vi "Harmonic Power.vi"(8 "error in (no error)":errorcluster, 10 "current spectra":T2(array[cluster]), 11 "voltage spectra":T2(array[cluster])) -> (0 "error out":errorcluster, 1 "total power value":T1, 2 "power values":T1[](array[typedef]), 3 "harmonic power values":T1[][](array[typedef]))   [LabVIEW 2013, in "NI_EP_Power Measurement.lvlib"]
doc: "Calculates the harmonic power values from the phase voltage spectra and the current spectra."
uses:
  <vilib>/addons/Electrical Power/Power Measurement/NI_EP_Power Measurement.lvlib
  <vilib>/addons/Electrical Power/Basic/Measurement/subVIs/basic_Power Value.ctl
  <vilib>/addons/Electrical Power/Basic/NI_EP_Basic.lvlib
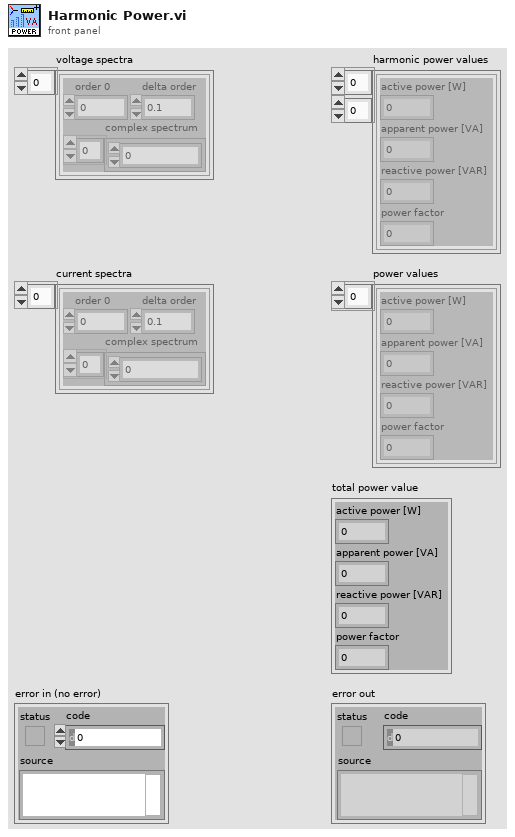
[diagram p1: front panel]
types:
  T1 = typedef "NI_EP_Basic.lvlib/basic_Power Value.ctl" = cluster{"active power [W]":dbl, "apparent power [VA]":dbl, "reactive power [VAR]":dbl, "power factor":dbl}
  T2 = cluster{"order 0":dbl, "delta order":dbl, "complex spectrum":cdb[]}[]
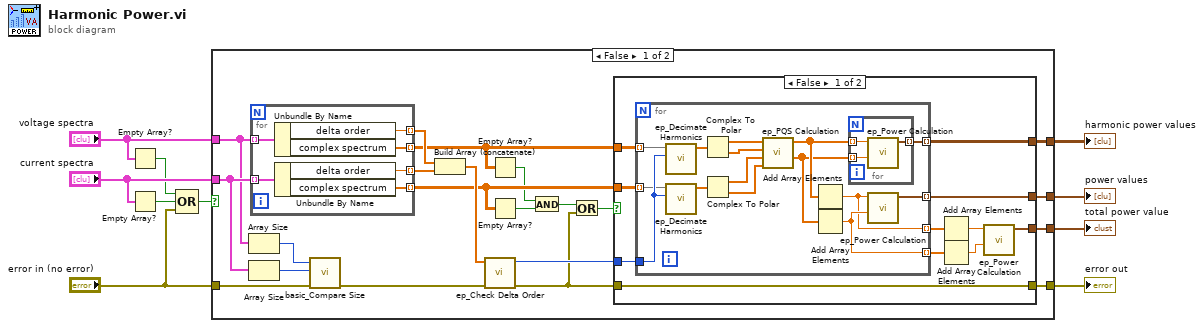
[diagram p0: block diagram]
diagram:
  n1 = Empty Array?(array="voltage spectra") -> (empty?=w3:bool)
  n2 = Empty Array?(array="current spectra") -> (empty?=w4:bool)
  n3 = Compound Arithmetic op=OR(w3, w4, "error in (no error)") -> (w2:bool)
  n4 = case shown="False" w2 {
    tunnel: [w31 _] -> w10
    tunnel: [w30 _] -> w9
    tunnel: [w29 _] -> w8
    tunnel: [w28 w68] -> w7
    tunnel: "current spectra" -> [w27 _]
    tunnel: "voltage spectra" -> [w26 _]
    tunnel: "error in (no error)" -> [w11 w68]
    frame False {
      n5 = Array Size(array=w26) -> (size(s)=w12:i32)
      n6 = Array Size(array=w27) -> (size(s)=w13:i32)
      n7 = for {
        tunnel: w27 -> [w36] mode=indexing
        tunnel: w26 -> [w37] mode=indexing
        tunnel: [w35] -> w24 mode=indexing
        tunnel: [w34] -> w22 mode=indexing
        tunnel: [w33] -> w21 mode=indexing
        tunnel: [w32] -> w25 mode=indexing
        n8 = Unbundle By Name(w37) -> ("delta order"=w35:dbl, "complex spectrum"=w34:cdb[])
        n9 = Unbundle By Name(w36) -> ("delta order"=w32:dbl, "complex spectrum"=w33:cdb[])
      }
      n10 = call <vilib>:"basic_Compare Size.vi"("error in (no error)"=w11, "size B"=w13, "size A"=w12) -> ("error out"=w14:errorcluster)  [unwired: 8 in]
      n11 = Build Array (concatenate)(w24, w25) -> (w23:dbl[])
      n12 = call <vilib>:"ep_Check Delta Order.vi"("error in (no error)"=w14, "delta order"=w23) -> ("error out"=w15:errorcluster, "cycles per block"=w20:i32)  [unwired: 8 in]
      n13 = Empty Array?(array=w22) -> (empty?=w18:bool)
      n14 = Empty Array?(array=w21) -> (empty?=w19:bool)
      n15 = And(x=w18, y=w19) -> (x .and. y?=w17:bool)
      n16 = Or(x=w17, y=w15) -> (x .or. y?=w16:bool)
      n17 = case shown="False" w16 {
        tunnel: [w48 _] -> w31
        tunnel: [w43 _] -> w29
        tunnel: [w42 _] -> w30
        tunnel: [w38 w67] -> w28
        tunnel: w22 -> [w41 _]
        tunnel: w21 -> [w40 _]
        tunnel: w20 -> [w39 _]
        tunnel: w15 -> [w38 w67]
        frame False {
          n18 = for {
            tunnel: w39 -> [w63]
            tunnel: [w56] -> w48 mode=indexing
            tunnel: [w53] -> w42 mode=indexing
            tunnel: [w52] -> w46 mode=indexing
            tunnel: [w51] -> w47 mode=indexing
            tunnel: w41 -> [w50] mode=indexing
            tunnel: w40 -> [w49] mode=indexing
            n19 = call <vilib>:"ep_Decimate Harmonics.vi"("decimation factor"=w63, "array in"=w50) -> ("decimated array"=w62:cdb[])  [unwired: 9 in]
            n20 = call <vilib>:"ep_Decimate Harmonics.vi"("decimation factor"=w63, "array in"=w49) -> ("decimated array"=w61:cdb[])  [unwired: 9 in]
            n21 = Complex To Polar(r * e^(i*theta)=w62) -> (r=w60:dbl[], theta=w57:dbl[])
            n22 = Complex To Polar(r * e^(i*theta)=w61) -> (r=w59:dbl[], theta=w58:dbl[])
            n23 = call <vilib>:"ep_PQS Calculation.vi"("I phase"=w58, "I magnitute"=w59, "U phase"=w57, "U magnitute"=w60) -> ("Q"=w54:dbl[], "P"=w55:dbl[])  [unwired: 5 in, 1 out]
            n24 = Add Array Elements(numeric array=w55) -> (sum=w51:dbl)
            n25 = Add Array Elements(numeric array=w54) -> (sum=w52:dbl)
            n26 = for {
              tunnel: w55 -> [w66] mode=indexing
              tunnel: [w65] -> w56 mode=indexing
              tunnel: w54 -> [w64] mode=indexing
              n27 = call <vilib>:"ep_Power Calculation.vi"("Q"=w64, "P"=w66) -> ("power values"=w65:T1)  [unwired: 9 in]
            }
            n28 = call <vilib>:"ep_Power Calculation.vi"("Q"=w52, "P"=w51) -> ("power values"=w53:T1)  [unwired: 9 in]
          }
          n29 = Add Array Elements(numeric array=w47) -> (sum=w45:dbl)
          n30 = Add Array Elements(numeric array=w46) -> (sum=w44:dbl)
          n31 = call <vilib>:"ep_Power Calculation.vi"("Q"=w44, "P"=w45) -> ("power values"=w43:T1)  [unwired: 9 in]
        }
        frame True {
        }
      }
    }
    frame True {
    }
  }
  "error out" <- w7
  "harmonic power values" <- w10
  "power values" <- w9
  "total power value" <- w8
